vi "Image.vi"(2 "XRef":refnum<vi>, 3 "State In":T1) -> (0 "Image":picture)   [LabVIEW 2017]
uses:
  <vilib>/UPVI/lvhdf5/xnodehelpers/State.ctl
  <vilib>/UPVI/lvhdf5/xnodehelpers/TermsPlus.ctl
  <vilib>/XNodeSupport/XNodeTerm3.ctl
  <vilib>/XNodeSupport/XNodeString.ctl
  <vilib>/XNodeSupport/XNodeVariant.ctl
  <vilib>/XNodeSupport/XNodeRect32.ctl
  <vilib>/XNodeSupport/XNodeInt.ctl
  <vilib>/XNodeSupport/XNodeBool.ctl
  <vilib>/XNodeSupport/XNodeTermDirection.ctl
  <vilib>/UPVI/lvhdf5/xnodehelpers/TermBehavior.ctl
  <vilib>/XNodeSupport/XNodeError3Array.ctl
  <vilib>/XNodeSupport/XNodeError3.ctl
  <vilib>/XNodeSupport/NI_XNodeSupport.lvlib
panel:
  # "LVHDF5 Toolkit\nCopyright (c) 2005-2013 by Jason D. Sommerville\nCopyright (c) 2014 by UPVI, LLC.\n\nThis use and distribution of this file is governed by the terms found in \nLICENSE.txt distributed with this toolkit and installed at\n <user.lib>\\_lvhdf5\\LICENSE.txt"
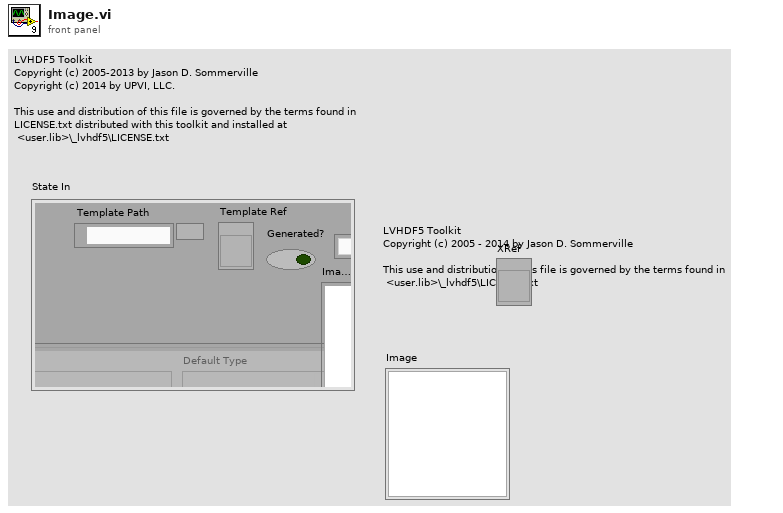
[diagram p1: front panel]
types:
  T1 = typedef "State.ctl" = cluster{"Template Path":path, "Template Ref":refnum<vi>, "Terms":T2[], "Display Name":string, "Image":picture, "Errors":T11, "Generated?":bool}
  T2 = typedef "TermsPlus.ctl" = cluster{"Term 3":T3, "Default Type":variant, "Behavior":T10, "Behavior Arg":string, "WiredResponse":bool, "Wired":enum16{"Unknown", "Unwired", "Wired"}}
  T3 = typedef "NI_XNodeSupport.lvlib/XNodeTerm3.ctl" = cluster{"Name":T4, "Id":T4, "Type":T5, "Bounds":T6, "Input?":T8, "Required?":T8, "Recommended?":T8, "Adaptive?":T8, "Hidden?":T8, "Direction":T9, "Break Wire?":T8}
  T4 = typedef "NI_XNodeSupport.lvlib/XNodeString.ctl" = string
  T5 = typedef "NI_XNodeSupport.lvlib/XNodeVariant.ctl" = variant
  T6 = typedef "NI_XNodeSupport.lvlib/XNodeRect32.ctl" = cluster{"Left":T7, "Top":T7, "Right":T7, "Bottom":T7}
  T7 = typedef "NI_XNodeSupport.lvlib/XNodeInt.ctl" = i32
  T8 = typedef "NI_XNodeSupport.lvlib/XNodeBool.ctl" = bool
  T9 = typedef "NI_XNodeSupport.lvlib/XNodeTermDirection.ctl" = enum32{"Auto", "Up", "Down", "Left", "Right", "Center"}
  T10 = typedef "TermBehavior.ctl" = enum16{"Normal", "Anything", "LVType", "Path or Ref", "Attr Name", "Attr Poly", "Elt Poly", "Dset Poly", "WDT Poly"}
  T11 = typedef "NI_XNodeSupport.lvlib/XNodeError3Array.ctl" = T12[]
  T12 = typedef "NI_XNodeSupport.lvlib/XNodeError3.ctl" = cluster{"Error":T4, "Details":T4, "Help File":T4, "Help Topic":T4}
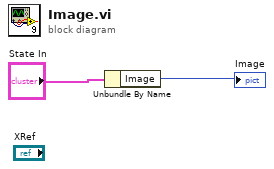
[diagram p0: block diagram]
diagram:
  n1 = Unbundle By Name("State In") -> ("Image"=→"Image":picture)
